vi "Add.vi"(8 "error in (no error)":errorcluster, 10 "Event Object":refnum<class "Event.lvclass">, 11 "EventBag in":refnum<class "EventBag.lvclass">) -> (0 "error out":errorcluster, 3 "EventBag out":refnum<class "EventBag.lvclass">)   [LabVIEW 2021, in "EventManagerLibrary.lvlib" / "EventBag.lvclass"]
uses:
  EventBag.lvclass
  EventObject/Event.lvclass
  EventBag.lvclass/EventBag.ctl
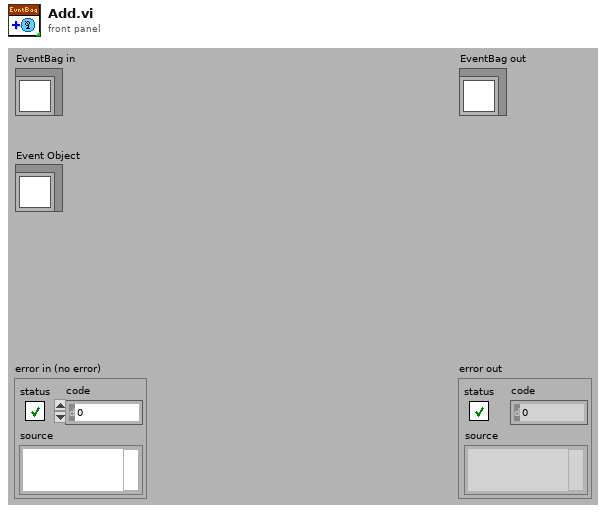
[diagram p1: front panel]
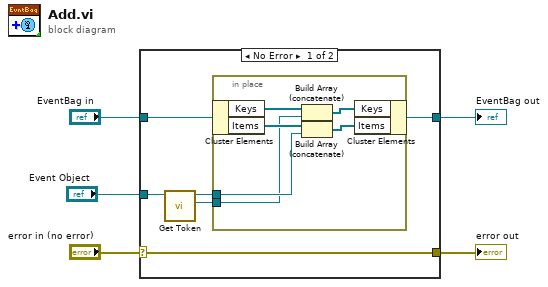
[diagram p0: block diagram]
diagram:
  n1 = case shown="No Error" "error in (no error)" {
    selector: "error in (no error)" -> [w11 w19]
    tunnel: [w11 w19] -> w4
    tunnel: [w8 w18] -> w2
    tunnel: "EventBag in" -> [w9 w18]
    tunnel: "Event Object" -> [w10 _]
    frame No Error {
      n2 = call-dynamic "Get Token.vi"("Event in"=w10) -> ("EventToken"=w6:refnum<class "EventToken.lvclass">, "Event out"=w7:refnum<class "Event.lvclass">)  [unwired: 1 in, 8 out]
      n3 = in-place {
        in-place-border: w7 -> [w13]
        in-place-border: w6 -> [w12]
        n4 = in-place-cluster #1(w9) -> ("Keys"=w17:refnum<class "EventToken.lvclass">[], "Items"=w15:refnum<class "Event.lvclass">[])
        n5 = Build Array (concatenate)(w17, w12) -> (w16:refnum<class "EventToken.lvclass">[])
        n6 = Build Array (concatenate)(w15, w13) -> (w14:refnum<class "Event.lvclass">[])
        n7 = in-place-cluster #1("Keys"=w16, "Items"=w14) -> (w8:refnum<class "EventBag.lvclass">)
      }
    }
    frame Error {
    }
  }
  "error out" <- w4
  "EventBag out" <- w2
